vi "readFromXML.vi"(8 "error in (no error)":errorcluster, 10 "XML in":string, 11 "TCSGuiderCommand.lvclass":refnum<class "TCSGuiderCommand.lvclass">) -> (0 "error out":errorcluster, 3 "TCSGuiderCommand.lvclass 2":refnum<class "TCSGuiderCommand.lvclass">)   [LabVIEW 2022 SP3, in "TCSDataDefinitions.lvlib" / "TCSGuiderCommand.lvlib" / "TCSGuiderCommand.lvclass"]
uses:
  TCSGuiderCommand.lvclass
  TCSCommand/TCSCommand/TCSCommand.lvclass
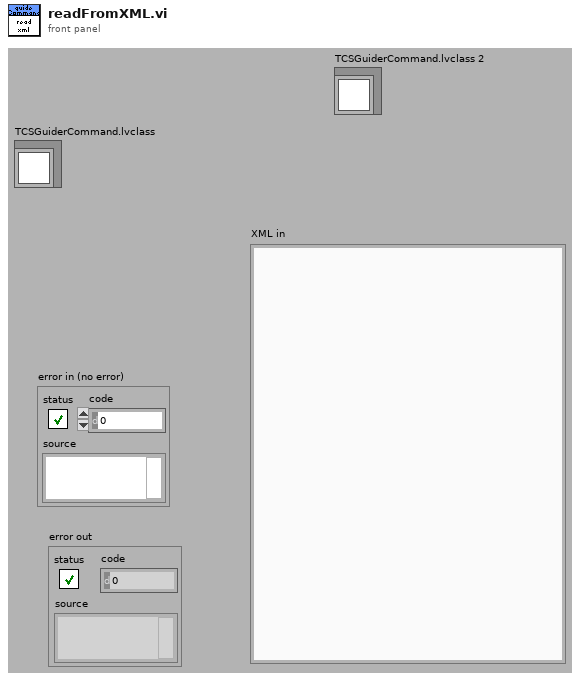
[diagram p1: front panel]
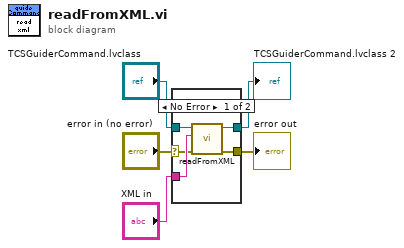
[diagram p0: block diagram]
diagram:
  n1 = case shown="No Error" "error in (no error)" {
    selector: "error in (no error)" -> [w9 w12]
    tunnel: [w8 w12] -> w4
    tunnel: [w6 w11] -> w1
    tunnel: "TCSGuiderCommand.lvclass" -> [w7 w11]
    tunnel: "XML in" -> [w10 _]
    frame No Error {
      n2 = call-parent "readFromXML.vi"("error in (no error)"=w9, "XML in"=w10, "TCSCommand in"=w7) -> ("error out"=w8:errorcluster, "TCSCommand out"=w6:refnum<class "TCSGuiderCommand.lvclass">)  [unwired: 7 in]
    }
    frame Error {
    }
  }
  "error out" <- w4
  "TCSGuiderCommand.lvclass 2" <- w1
